vi "HAPS_LoadTable_SetBeam_Manual_Selected_Leo.vi"() -> ()   [LabVIEW 2023, in "HAPS.lvlib"]
uses:
  HAPS.lvlib
  set_ele.ctl
  HAPS_SerialPort.ctl
  HAPS_MCU_ELE_Func.ctl
  <vilib>/Utility/file.llb/Read Delimited Spreadsheet (string).vi
  R_S/R_S.lvlib
panel:
  in  "Preamp_ch":i32
  out "error IO":errorcluster
  out "Err_code":i32
  out "status":bool
  in  "offset?":bool
  in  "simu.?":bool
  in  "set_ele":T1={"ch"=0, "chain_id"=0, "group"=0, "array_id"=0, "ele_phase"=0, "ele_gain"=35, "com_gain"=17, "pd_range"=0}
  in  "ele_gain":i32=35
  in  "BFIC_id?":i32
  in  "Group?":i32
  in  "sys reboot?":bool=TRUE
  in  "VISA resource name":refnum<visa-resource-name>="COM1"
  in  "file path":path=path "C:/Users/Vince_Wu/Desktop/HAPS_PIC/20260606/Tx/No_1_Tx_all/HAPS_Phase_Sweep_Tx_MCU0_COM1_NO1_H_ALL_20250606_204323_14_Inphase.csv"
  out "Remaining quantity":i32
  out "ele phase":i32
  out "ele gain":i32
  out "channel":i32
  out "chain ID":i32
  out "group":i32
  out "array id":i32
  # "HAPS 24x24 Setting Manual In-Phase : \n                                                   One BFIC Leo"
  # "Tx:35\nRx:22"
  # "Not using!!!!!!!!!!!!!!!!!!!!!!!!!!!!!!!!!!!!!!!!"
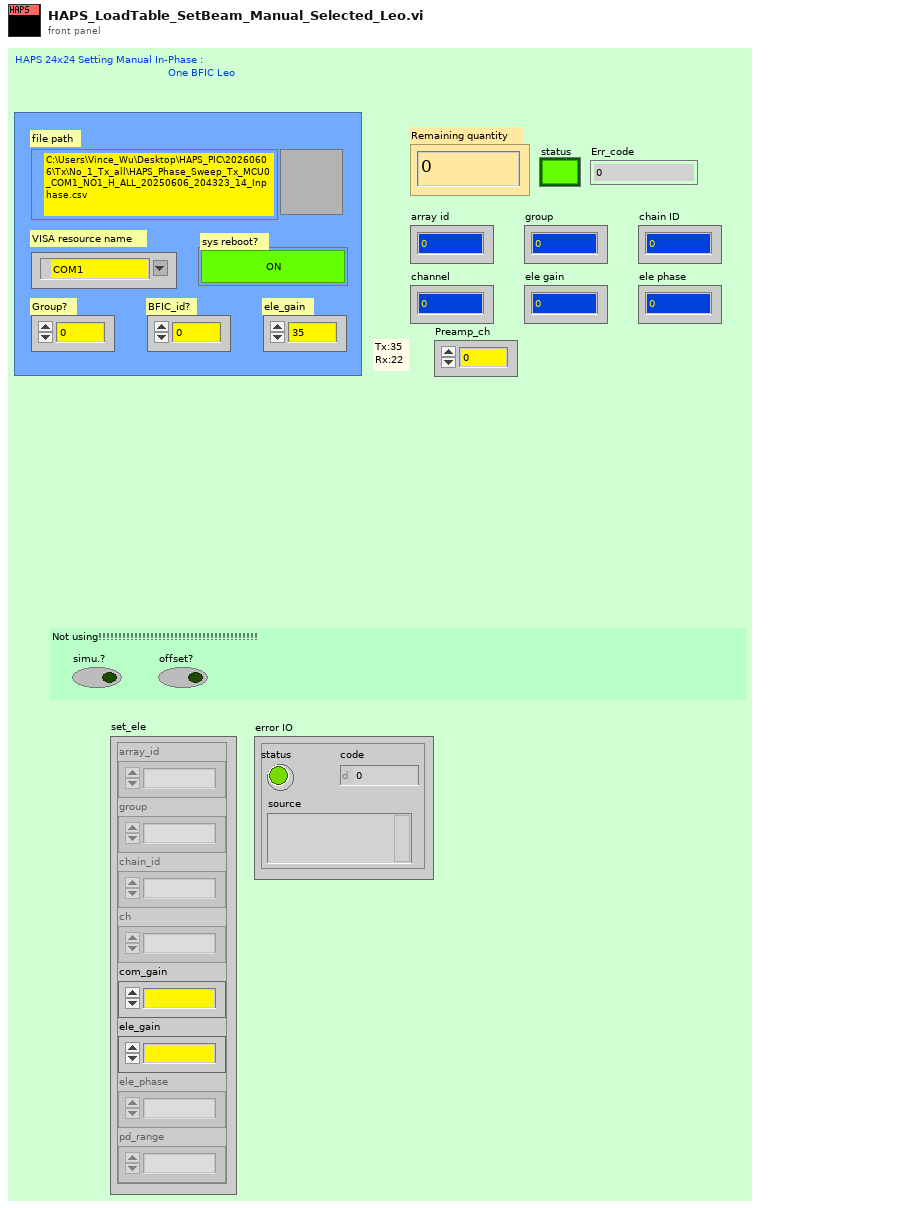
[diagram p1: front panel]
types:
  T1 = typedef "HAPS.lvlib/set_ele.ctl" = cluster{"ch":i32, "chain_id":i32, "group":i32, "array_id":i32, "ele_phase":i32, "ele_gain":i32, "com_gain":i32, "pd_range":i32}
  T2 = typedef "HAPS.lvlib/HAPS_SerialPort.ctl" = enum16{"Init", "Close", "CMD", "Flush"}
  T3 = typedef "HAPS.lvlib/HAPS_MCU_ELE_Func.ctl" = enum16{"array_init", "set_com_gain", "set_ch_gain_phase", "set_pd_range", "get_preamp_temp", "get_bfic_temp", "get_tx_pd", "ch_on", "ch_on_2", "ch_ctrl_all", "array_ctrl_src"}
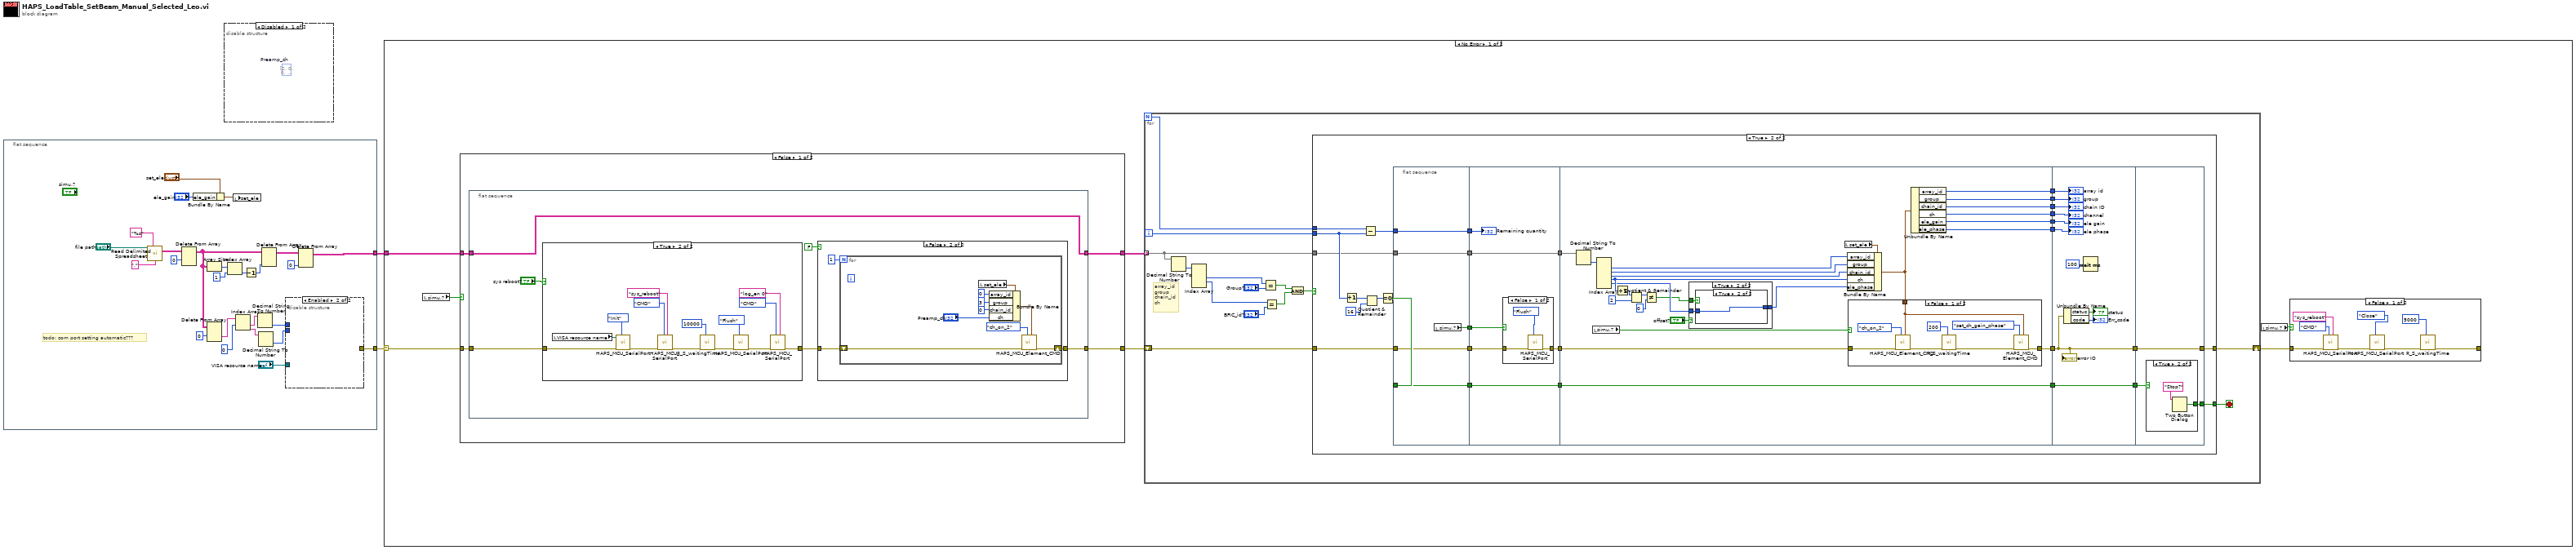
[diagram p0: block diagram]
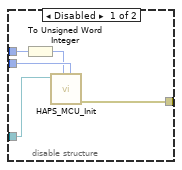
[diagram p2: hidden frame]
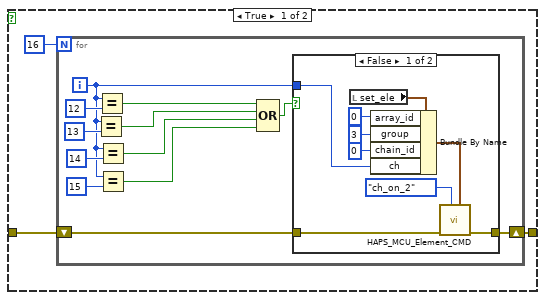
[diagram p5: hidden frame]
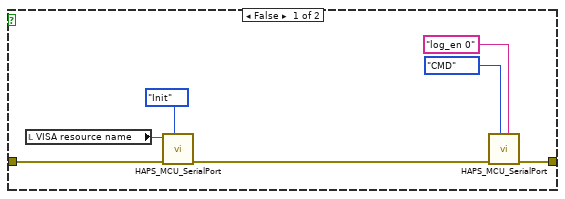
[diagram p7: hidden frame]
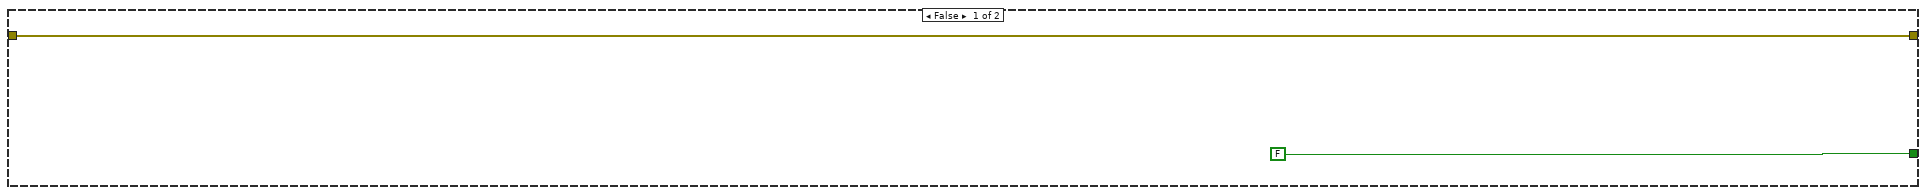
[diagram p9: hidden frame]
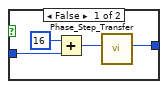
[diagram p12: hidden frame]
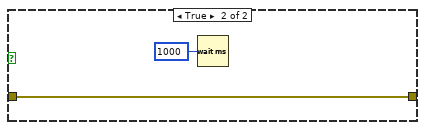
[diagram p13: hidden frame]
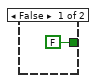
[diagram p14: hidden frame]
diagram:
  n1 = flat-sequence {
    tunnel: [w19] -> w2
    tunnel: [w6] -> w1
    frame #0 {
      # "todo: com port setting automatic???"
      n2 = call-poly <vilib>:"Read Delimited Spreadsheet.vi"("file path (dialog if empty)"="file path", "format (%s)"="%s" ("format (%.3f)"), "delimiter (\\t)"="," ("delimiter (\\t)")) -> ("all rows"=w25:string[][])  [unwired: 7 in, 5 out]
      n3 = Delete From Array(array=w25, index (row)=0) -> (array with subset deleted=w15:string[][])  [unwired: 2 in, 1 out]
      n4 = Bundle By Name(cluster="set_ele", "ele_gain"="ele_gain") -> (w3:T1)
      n5 = Array Size(array=w15) -> (size(s)=w23:i32[])
      n6 = Delete From Array(array=w15, index (row)=0) -> (deleted portion=w14:string[])  [unwired: 2 in, 1 out]
      n7 = Index Array(array=w23, index=1) -> (element=w20:i32)
      n8 = local write "set_ele"(w3) -> ()
      n9 = Index Array(array=w14, index #1=0 ("index")) -> (element #1=w13:string, element #2=w12:string)  [unwired: 1 in]
      n10 = Decrement(x=w20) -> (x-1=w22:i32)
      n11 = Decimal String To Number(string=w13) -> (number=w9:i32)  [unwired: 2 in, 1 out]
      n12 = Decimal String To Number(string=w12) -> (number=w8:i32)  [unwired: 2 in, 1 out]
      n13 = Delete From Array(array=w15, index (col)=w22) -> (array with subset deleted=w18:string[][])  [unwired: 2 in, 1 out]
      n14 = disable-structure shown="Enabled" {
        disable-tunnel: [w32 _] -> w19
        disable-tunnel: w9 -> [w31 _]
        disable-tunnel: w8 -> [w30 _]
        disable-tunnel: "VISA resource name" -> [w29 _]
        frame Disabled {
          n15 = To Unsigned Word Integer(number=w31) -> (unsigned 16bit integer=w28:u16)
          n16 = call "HAPS_MCU_Init.vi"("array_id"=w30, "Tx/Rx"=w28, "VISA resource name"=w29) -> ("error out"=w32:errorcluster)  [unwired: 8 in]
        }
        frame Enabled {
        }
      }
      n17 = Delete From Array(array=w18, index (col)=0 ("index (row)")) -> (array with subset deleted=w6:string[][])  [unwired: 2 in, 1 out]
    }
  }
  n18 = disable-structure shown="Disabled" {
    frame Disabled {
      (unwired) i32[][] [[2, 0, 0, 8, 8, 10, 11, 9, 9, 1, 1, 3], [3, 1, 1, 9, 9, 11, 13, 15, 15, 7, 7, 5], [5, 7, 7, 15, 15, 13, 14, 14, 6, 6, 4, 12]]  # Preamp_ch
    }
    frame Enabled {
    }
  }
  n19 = case shown="No Error" w2 {
    selector: w2 -> [w37 _]
    tunnel: w1 -> [w39 _]
    frame No Error {
      n20 = local read "simu.?"() -> (w35:bool)
      n21 = case shown="False" w35 {
        tunnel: w39 -> [w52 w118]
        tunnel: [w51 w118] -> w38
        tunnel: w37 -> [w50 w117]
        tunnel: [w49 w117] -> w36
        frame False {
          n22 = flat-sequence {
            tunnel: w52 -> [w58]
            tunnel: [w58] -> w51
            tunnel: w50 -> [w56]
            tunnel: [w57] -> w49
            frame #0 {
              n23 = case shown="True" "sys reboot?" {
                tunnel: w56 -> [w100 w114]
                tunnel: [w98 w112] -> w55
                frame False {
                  n24 = local read "VISA resource name"() -> (w96:refnum<visa-resource-name>)
                  n25 = call "HAPS_MCU_SerialPort.vi"("HAPS_SerialPort_Func"=HAPS_SerialPort."Init", "error in"=w100, "VISA resource name"=w96) -> ("error out"=w97:errorcluster)  [unwired: 6 in, 2 out]
                  n26 = call "HAPS_MCU_SerialPort.vi"("Command"="log_en 0", "HAPS_SerialPort_Func"=enum16{"Init", "Close", "CMD"}."CMD" ("HAPS_SerialPort"), "error in"=w97) -> ("error out"=w98:errorcluster)  [unwired: 6 in, 2 out]
                }
                frame True {
                  n27 = local read "VISA resource name"() -> (w103:refnum<visa-resource-name>)
                  n28 = call "HAPS_MCU_SerialPort.vi"("HAPS_SerialPort_Func"=HAPS_SerialPort."Init", "error in"=w114, "VISA resource name"=w103) -> ("error out"=w109:errorcluster)  [unwired: 6 in, 2 out]
                  n29 = call "HAPS_MCU_SerialPort.vi"("Command"="sys_reboot", "HAPS_SerialPort_Func"=enum16{"Init", "Close", "CMD"}."CMD" ("HAPS_SerialPort"), "error in"=w109) -> ("error out"=w108:errorcluster)  [unwired: 6 in, 2 out]
                  n30 = call "R_S_waitingTime.vi"("Waiting Time(ms)"=u32 10000, "error in"=w108) -> ("error out"=w106:errorcluster)  [unwired: 9 in]
                  n31 = call "HAPS_MCU_SerialPort.vi"("HAPS_SerialPort_Func"=HAPS_SerialPort."Flush", "error in"=w106) -> ("error out"=w104:errorcluster)  [unwired: 7 in, 2 out]
                  n32 = call "HAPS_MCU_SerialPort.vi"("Command"="log_en 0", "HAPS_SerialPort_Func"=enum16{"Init", "Close", "CMD"}."CMD" ("HAPS_SerialPort"), "error in"=w104) -> ("error out"=w112:errorcluster)  [unwired: 6 in, 2 out]
                }
              }
              n33 = case shown="False" FALSE {
                tunnel: [w60 w85] -> w57
                tunnel: w55 -> [w59 w84]
                frame True {
                  n34 = for {
                    N: 16 -> [_]
                    shift-right: [w72] -> w60
                    shift-left: w59 -> [w73]
                    i -> [w63]
                    n35 = Equal?(x=w63, y=13) -> (x = y?=w67:bool)
                    n36 = Equal?(x=w63, y=12) -> (x = y?=w71:bool)
                    n37 = Equal?(x=w63, y=14) -> (x = y?=w65:bool)
                    n38 = Equal?(x=w63, y=15) -> (x = y?=w62:bool)
                    n39 = Compound Arithmetic op=OR(w71, w67, w65, w62) -> (w68:bool)
                    n40 = case shown="False" w68 {
                      tunnel: w73 -> [w76 w83]
                      tunnel: [w75 w83] -> w72
                      tunnel: w63 -> [w74 _]
                      frame False {
                        n41 = local read "set_ele"() -> (w78:T1)
                        n42 = Bundle By Name(cluster=w78, "array_id"=0, "group"=3, "chain_id"=0, "ch"=w74) -> (w79:T1)
                        n43 = call "HAPS_MCU_Element_CMD.vi"("set_ele"=w79, "HAPS_MCU_ELE_Func."=HAPS_MCU_ELE_Func."ch_on_2", "error in"=w76) -> ("error out"=w75:errorcluster)  [unwired: 7 in, 1 out]
                      }
                      frame True {
                      }
                    }
                  }
                }
                frame False {
                  n44 = for {
                    N: 1 -> [_]
                    shift-right: [w94] -> w85
                    shift-left: w84 -> [w95]
                    n45 = local read "set_ele"() -> (w89:T1)
                    n46 = Bundle By Name(cluster=w89, "array_id"=0, "group"=3, "chain_id"=0, "ch"="Preamp_ch") -> (w90:T1)
                    n47 = call "HAPS_MCU_Element_CMD.vi"("set_ele"=w90, "HAPS_MCU_ELE_Func."=HAPS_MCU_ELE_Func."ch_on_2", "error in"=w95) -> ("error out"=w94:errorcluster)  [unwired: 7 in, 1 out]
                  }
                }
              }
            }
          }
        }
        frame True {
        }
      }
      n48 = for {
        N -> [w130]
        tunnel: w38 -> [w127] mode=indexing
        shift-right: [w132] -> w33
        shift-left: w36 -> [w131]
        i -> [w129]
        stop <- w126 stop-if-true
        # "array_id\ngroup\nchain_id\nch"
        n49 = Decimal String To Number(string=w127) -> (number=w128:i32[])  [unwired: 2 in, 1 out]
        n50 = Index Array(array=w128) -> (element #2=w125:i32, element #3=w123:i32)  [unwired: 4 in, 2 out]
        n51 = Equal?(x=w125, y="Group?") -> (x = y?=w121:bool)
        n52 = Equal?(x=w123, y="BFIC_id?") -> (x = y?=w120:bool)
        n53 = Compound Arithmetic op=AND(w121, w120) -> (w119:bool)
        n54 = case shown="True" w119 {
          tunnel: [w133 w146] -> w132
          tunnel: w131 -> [w133 w145]
          tunnel: w130 -> [_ w144]
          tunnel: w129 -> [_ w143]
          tunnel: w127 -> [_ w142]
          tunnel: [FALSE ("T button?") w136] -> w126
          frame False {
          }
          frame True {
            n55 = Increment(x=w143) -> (x+1=w140:i32)
            n56 = Subtract(x=w144, y=w143) -> (x-y=w141:i32)
            n57 = Quotient & Remainder(x=w140, y=16) -> (x-y*floor(x/y)=w138:i32)  [unwired: 1 out]
            n58 = Equal To 0?(x=w138) -> (x = 0?=w137:bool)
            n59 = flat-sequence {
              tunnel: w141 -> [w166]
              tunnel: w145 -> [w167]
              tunnel: w142 -> [w168]
              tunnel: [w168] -> w163
              tunnel: [w167] -> w162
              tunnel: [w166] -> w161
              tunnel: w137 -> [w165]
              tunnel: [w165] -> w160
              tunnel: [w164] -> w135
              tunnel: [w173] -> w159
              tunnel: [w172] -> w158
              tunnel: w163 -> [w173]
              tunnel: w162 -> [w171]
              tunnel: w161 -> [w174]
              tunnel: w160 -> [w170]
              tunnel: [w170] -> w157
              tunnel: w135 -> [w169]
              tunnel: w159 -> [w204]
              tunnel: w158 -> [w202]
              tunnel: [w190] -> w156
              tunnel: [w200] -> w155
              tunnel: [w199] -> w154
              tunnel: [w198] -> w153
              tunnel: [w197] -> w152
              tunnel: [w196] -> w151
              tunnel: [w195] -> w150
              tunnel: w157 -> [w191]
              tunnel: [w191] -> w149
              tunnel: w156 -> [w226]
              tunnel: w155 -> [w234]
              tunnel: w154 -> [w233]
              tunnel: w153 -> [w232]
              tunnel: w152 -> [w231]
              tunnel: w151 -> [w230]
              tunnel: w150 -> [w229]
              tunnel: [w226] -> w148
              tunnel: w149 -> [w227]
              tunnel: [w227] -> w147
              tunnel: w148 -> [w237]
              tunnel: w147 -> [w236]
              tunnel: [w237] -> w146
              tunnel: [w235] -> w136
              frame #0 {
                n60 = local read "simu.?"() -> (w164:bool)
              }
              frame #1 {
                n61 = case shown="False" w169 {
                  tunnel: [w177 w178] -> w172
                  tunnel: w171 -> [w176 w178]
                  frame False {
                    n62 = call "HAPS_MCU_SerialPort.vi"("HAPS_SerialPort_Func"=HAPS_SerialPort."Flush", "error in"=w176) -> ("error out"=w177:errorcluster)  [unwired: 7 in, 2 out]
                  }
                  frame True {
                  }
                }
                "Remaining quantity" <- w174
              }
              frame #2 {
                n63 = Decimal String To Number(string=w204) -> (number=w203:i32[])  [unwired: 2 in, 1 out]
                n64 = local read "simu.?"() -> (w189:bool)
                n65 = Index Array(array=w203) -> (element #1=w201:i32, element #2=w194:i32, element #3=w193:i32, element #4=w187:i32, element #5=w183:i32)  [unwired: 6 in, 1 out]
                n66 = Increment(x=w187) -> (x+1=w179:i32)
                n67 = Quotient & Remainder(x=w179, y=2) -> (x-y*floor(x/y)=w185:i32)  [unwired: 1 out]
                n68 = Not Equal?(x=w185, y=0) -> (x != y?=w182:bool)
                n69 = case shown="True" "offset?" {
                  tunnel: w183 -> [w205 w208]
                  tunnel: w182 -> [_ w207]
                  tunnel: [w205 w206] -> w181
                  frame False {
                  }
                  frame True {
                    n70 = case shown="True" w207 {
                      tunnel: w208 -> [w212 w213]
                      tunnel: [w209 w213] -> w206
                      frame False {
                        n71 = Add(x=16, y=w212) -> (x+y=w210:i32)
                        n72 = call "Phase_Step_Transfer.vi"("Input_Phase_Step"=w210) -> ("Output_Phase_Step"=w209:i32)  [unwired: 10 in]
                      }
                      frame True {
                      }
                    }
                  }
                }
                n73 = local read "set_ele"() -> (w192:T1)
                n74 = Bundle By Name(cluster=w192, "array_id"=w201, "group"=w194, "chain_id"=w193, "ch"=w187, "ele_phase"=w181) -> (w188:T1)
                n75 = case shown="False" w189 {
                  tunnel: w202 -> [w221 w223]
                  tunnel: w188 -> [w220 _]
                  tunnel: [w219 w223] -> w190
                  frame False {
                    n76 = call "HAPS_MCU_Element_CMD.vi"("set_ele"=w220, "HAPS_MCU_ELE_Func."=HAPS_MCU_ELE_Func."ch_on_2", "error in"=w221) -> ("error out"=w215:errorcluster)  [unwired: 7 in, 1 out]
                    n77 = call "R_S_waitingTime.vi"("Waiting Time(ms)"=u32 200, "error in"=w215) -> ("error out"=w214:errorcluster)  [unwired: 9 in]
                    n78 = call "HAPS_MCU_Element_CMD.vi"("set_ele"=w220, "HAPS_MCU_ELE_Func."=HAPS_MCU_ELE_Func."set_ch_gain_phase", "error in"=w214) -> ("error out"=w219:errorcluster)  [unwired: 7 in, 1 out]
                  }
                  frame True {
                    n79 = Wait (ms)(milliseconds to wait=u32 1000) -> ()  [unwired: 1 out]
                  }
                }
                n80 = Unbundle By Name(w188) -> ("array_id"=w200:i32, "group"=w199:i32, "chain_id"=w198:i32, "ch"=w197:i32, "ele_gain"=w196:i32, "ele_phase"=w195:i32)
              }
              frame #3 {
                n81 = Unbundle By Name(w226) -> ("status"=→"status":bool, "code"=→"Err_code":i32)
                n82 = Wait (ms)(milliseconds to wait=u32 100) -> ()  [unwired: 1 out]
                "group" <- w233
                "chain ID" <- w232
                "channel" <- w231
                "ele gain" <- w230
                "ele phase" <- w229
                "array id" <- w234
                "error IO" <- w226
              }
              frame #4 {
                n83 = case shown="True" w236 {
                  tunnel: [FALSE ("T button?") w239] -> w235
                  frame False {
                  }
                  frame True {
                    n84 = Two Button Dialog(message="Stop?") -> (T button?=w239:bool)  [unwired: 2 in]
                  }
                }
              }
            }
          }
        }
      }
      n85 = local read "simu.?"() -> (w34:bool)
      n86 = case shown="False" w34 {
        tunnel: [w40 w48] -> _
        tunnel: w33 -> [w47 w48]
        frame False {
          n87 = call "HAPS_MCU_SerialPort.vi"("Command"="sys_reboot", "HAPS_SerialPort_Func"=enum16{"Init", "Close", "CMD"}."CMD" ("HAPS_SerialPort"), "error in"=w47) -> ("error out"=w43:errorcluster)  [unwired: 6 in, 2 out]
          n88 = call "HAPS_MCU_SerialPort.vi"("HAPS_SerialPort_Func"=HAPS_SerialPort."Close", "error in"=w43) -> ("error out"=w41:errorcluster)  [unwired: 7 in, 2 out]
          n89 = call "R_S_waitingTime.vi"("Waiting Time(ms)"=u32 5000, "error in"=w41) -> ("error out"=w40:errorcluster)  [unwired: 9 in]
        }
        frame True {
        }
      }
    }
    frame Error {
    }
  }
